vi "WILT Type Conv - U8 to Status.vi"(10 "Byte Val":u8) -> (2 "Status":T1)   [LabVIEW 2016]
uses:
  Type Definitions/WILT Dryer Status Ctrl.ctl
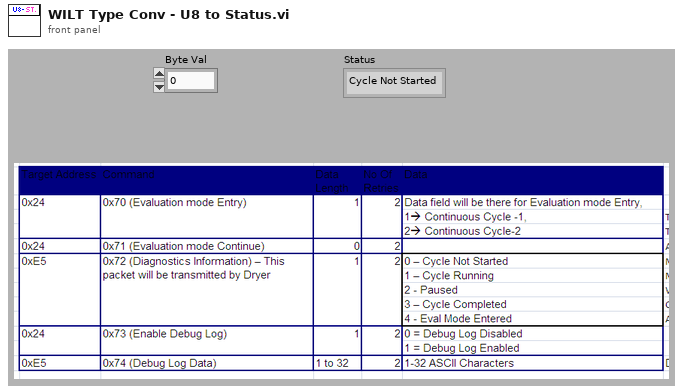
[diagram p1: front panel]
types:
  T1 = typedef "WILT Dryer Status Ctrl.ctl" = enum16{"Cycle Not Started", "Cycle Running", "Paused", "Cycle Completed", "Eval Mode Entered", "Err", "Pause (No GEA2)"}
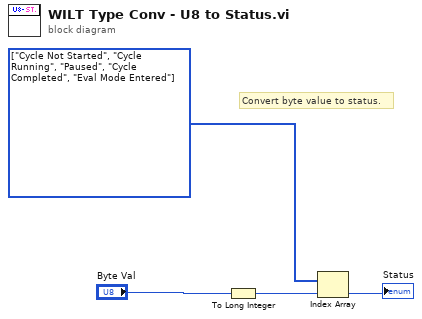
[diagram p0: block diagram]
diagram:
  w4 = T1[] [enum."Cycle Not Started", enum."Cycle Running", enum."Paused", enum."Cycle Completed", enum."Eval Mode Entered"] items=["Cycle Not Started", "Cycle Running", "Paused", "Cycle Completed", "Eval Mode Entered", "Err", "Pause (No GEA2)"]
  # "Convert byte value to status."
  n1 = To Long Integer(number="Byte Val") -> (32bit integer=w1:i32)
  n2 = Index Array(array=w4, index=w1) -> (element=→"Status":T1)
